vi "后台任务主调VI.vi"() -> ()   [LabVIEW 2013]
uses:
  <resource>/importtools/Common/Event/NISAST Event.lvclass
panel:
  out "ChannelA Data":dbl
  out "ChannelB Data":dbl
  in  "停止后台任务":bool
  in  "启动后台任务":bool
  in  "停止":bool
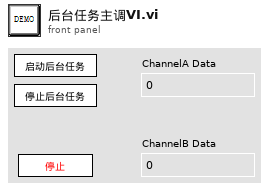
[diagram p1: front panel]
types:
  T1 = enum32{"Bad", "Idle", "Run top level", "Running"}
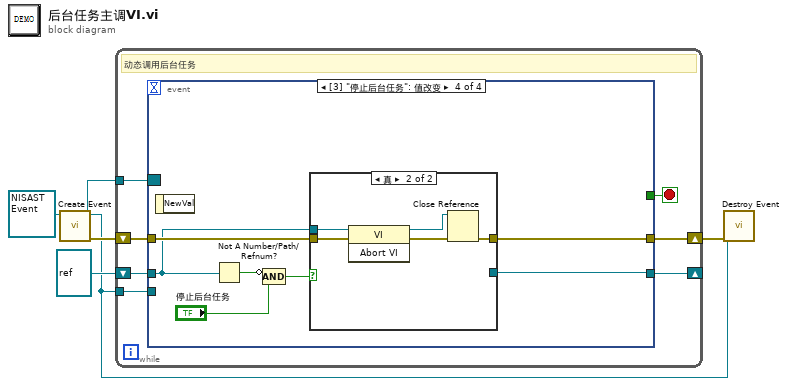
[diagram p0: block diagram]
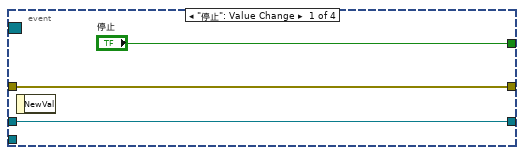
[diagram p2: hidden frame]
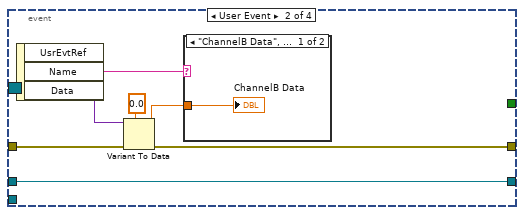
[diagram p3: hidden frame]
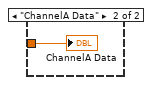
[diagram p4: hidden frame]
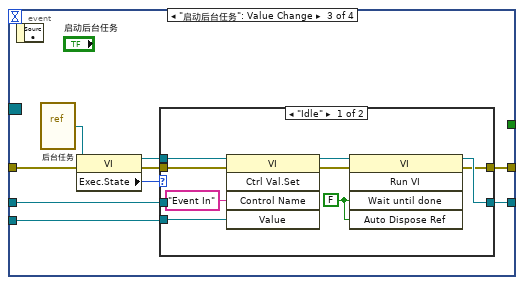
[diagram p5: hidden frame]
diagram:
  n1 = call-dynamic "Create Event.vi"("Event in"=refnum<class "NISAST Event.lvclass"> refnum) -> ("error out"=w6:errorcluster, "Event Registration Refnum"=w5:refnum<event-registration>, "Event out"=w2:refnum<class "NISAST Event.lvclass">)  [unwired: 8 in]
  n2 = while {
    shift-right: [w10] -> w3
    shift-left: w6 -> [w11]
    tunnel: w2 -> [w9]
    tunnel: w5 -> [w12]
    shift-right: [w8] -> _
    shift-left: refnum<vi> refnum -> [w7]
    stop <- w13 stop-if-true
    # "动态调用后台任务"
    n3 = event shown="[3] \"停止后台任务\": 值改变" {
      selector: w12 -> [_ _ _ _]
      dyn-events: _ -> [_ _ _ _]
      timeout: _ -> [_ _ _ _]
      tunnel: ["停止" _ _ _] -> w13
      tunnel: w11 -> [w15 w18 w27 w52]
      tunnel: [w15 w17 w28 w51] -> w10
      tunnel: w9 -> [_ _ w30 _]
      tunnel: [w14 w19 w29 w50] -> w8
      tunnel: w7 -> [w14 w19 w26 w49]
      event "停止": Value Change {
        n4 = event-data() -> ()  [unwired: 1 in, 1 out]
      }
      event User Event {
        n5 = event-data() -> ("Name"=w21:string, "Data"=w23:variant)  [unwired: 1 in, 1 out]
        n6 = Variant To Data(error in=w18, type=0.0, Variant=w23) -> (data=w20:dbl, error out=w17:errorcluster)
        n7 = case shown="\"ChannelB Data\", 默认" w21 {
          tunnel: w20 -> [w24 w25]
          frame "ChannelB Data", Default {
            "ChannelB Data" <- w24
          }
          frame "ChannelA Data" {
            "ChannelA Data" <- w25
          }
        }
      }
      event "启动后台任务": Value Change {
        n8 = event-data() -> ()  [unwired: 1 in, 1 out]
        n9 = vi-ref "后台任务.vi"() -> (w34:refnum<vi>)
        n10 = property class="VI"(reference=w34, error in=w27) -> (reference out=w32:refnum<vi>, error out=w31:errorcluster, "Exec.State"=w33:T1)
        n11 = case shown="\"Idle\"" w33 {
          tunnel: w32 -> [w43 _]
          tunnel: w31 -> [w42 w45]
          tunnel: w30 -> [w41 _]
          tunnel: [w37 w44] -> w29
          tunnel: [w36 w45] -> w28
          tunnel: w26 -> [_ w44]
          frame "Idle" {
            w35 = FALSE ("结束前等待")
            n12 = invoke class="VI" method="Ctrl Val.Set"(reference=w43, error in=w42, "Control Name"="Event In" ("控件名"), "Value"=w41) -> (reference out=w39:refnum<vi>, error out=w38:errorcluster)  [unwired: 1 in, 3 out]
            n13 = invoke class="VI" method="Run VI"(reference=w39, error in=w38, "Wait until done"=w35, "Auto Dispose Ref"=w35) -> (reference out=w37:refnum<vi>, error out=w36:errorcluster)  [unwired: 1 in, 3 out]
          }
          frame "Running", Default {
          }
        }
      }
      event "停止后台任务": Value Change {
        n14 = event-data() -> ()  [unwired: 1 in, 1 out]
        n15 = Not A Number/Path/Refnum?(number/path/refnum=w49) -> (NaN/Path/Refnum?=w46:bool)
        n16 = Compound Arithmetic op=AND(invert w46, "停止后台任务") -> (w48:bool)
        n17 = case shown="真" w48 {
          tunnel: w49 -> [w53 w59]
          tunnel: w52 -> [w54 w58]
          tunnel: [w54 w55] -> w51
          tunnel: [w53 _] -> w50
          frame False {
          }
          frame True {
            n18 = invoke class="VI" method="Abort VI"(reference=w59, error in=w58) -> (reference out=w57:refnum<vi>, error out=w56:errorcluster)  [unwired: 1 in, 1 out]
            n19 = Close Reference(reference=w57, error in (no error)=w56) -> (error out=w55:errorcluster)
          }
        }
      }
    }
  }
  n20 = call-dynamic "Destroy Event.vi"("error in (no error)"=w3, "Event in"=w2) -> ()  [unwired: 8 in, 2 out]
